vi "Experiment header-Maintenance.vi"(8 "error in (no error)":errorcluster, 9 "<Valid parameter names>":string[](array[string]), 10 "section":string, 11 "Experiment header file ref in":T1) -> (0 "error out":errorcluster, 3 "Experiment header file ref":T1)   [LabVIEW 2013]
uses:
  <vilib>/Utility/config.llb/Config Data RefNum.ctl
  <vilib>/Utility/config.llb/NI_LVConfig.lvlib
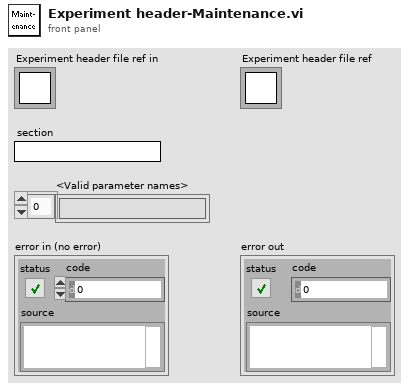
[diagram p1: front panel]
types:
  T1 = typedef "NI_LVConfig.lvlib/Config Data RefNum.ctl" = refnum<k1>
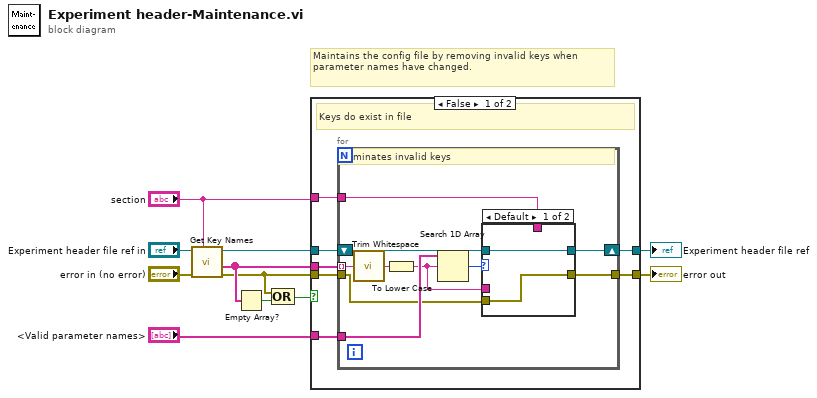
[diagram p0: block diagram]
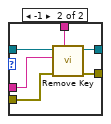
[diagram p2: hidden frame]
diagram:
  # "Maintains the config file by removing invalid keys when parameter names have changed."
  n1 = call <vilib>:"Get Key Names.vi"("section"="section", "error in (no error)"="error in (no error)", "refnum"="Experiment header file ref in") -> ("error out"=w7:errorcluster, "key names"=w10:string[], "refnum out"=w3:T1)  [unwired: 5 in, 1 out]
  n2 = Empty Array?(array=w10) -> (empty?=w5:bool)
  n3 = Compound Arithmetic op=OR(w7, w5) -> (w6:bool)
  n4 = case shown="False" w6 {
    tunnel: "<Valid parameter names>" -> [w18 _]
    tunnel: w10 -> [w17 _]
    tunnel: w3 -> [w16 w38]
    tunnel: [w15 w38] -> w4
    tunnel: w7 -> [w14 w37]
    tunnel: [w13 w37] -> w8
    tunnel: "section" -> [w12 _]
    frame False {
      # "Keys do exist in file"
      n5 = for {
        tunnel: w18 -> [w28]
        tunnel: w17 -> [w21] mode=indexing
        shift-right: [w26] -> w15
        shift-left: w16 -> [w27]
        tunnel: w14 -> [w25]
        tunnel: [w24] -> w13
        tunnel: w12 -> [w23]
        # "Eliminates invalid keys"
        n6 = call <vilib>:"Trim Whitespace.vi"("string"=w21) -> ("trimmed string"=w22:string)  [unwired: 1 in]
        n7 = To Lower Case(string=w22) -> (all lower case string=w20:string)
        n8 = Search 1D Array(1D array=w28, element=w20) -> (index of element=w19:i32)  [unwired: 1 in]
        n9 = case shown="Default" w19 {
          tunnel: w27 -> [w30 w36]
          tunnel: [w30 w35] -> w26
          tunnel: w25 -> [w29 w34]
          tunnel: [w29 w33] -> w24
          tunnel: w23 -> [_ w32]
          tunnel: w20 -> [_ w31]
          frame Default {
          }
          frame -1 {
            n10 = call <vilib>:"Remove Key.vi"("section"=w32, "error in (no error)"=w34, "key"=w31, "refnum"=w36) -> ("error out"=w33:errorcluster, "refnum out"=w35:T1)  [unwired: 5 in, 1 out]
          }
        }
      }
    }
    frame True {
      # "No keys found, or Error"
    }
  }
  "error out" <- w8
  "Experiment header file ref" <- w4
